vi "MT Generate Bits (Galois, PN Order).vi"(0 "total bits (128)":i32=128, 7 "PN sequence order (9)":i32=9, 9 "seed in (0xD6BF7DF2)":i32=-692093454 format="%.0x", 11 "error in (no error)":errorcluster, 13 "reset? (T)":bool=TRUE) -> (4 "output bit stream":i8[](array[numeric]), 10 "seed out":i32 format="%.0x", 15 "error out":errorcluster)   [LabVIEW 2020, in "niDMT.lvlib"]
doc: "This polymorphic instance generates Galois pseudonoise (PN) bit sequences. The VI repeats the selected pattern until it generates number of total bits that you specify. Use this instance to specify a PN sequence order based on which the VI selects a primitive polynomial that returns an m-sequence."
uses:
  <vilib>/addons/Modulation/niDMT.lvlib
  <vilib>/addons/Modulation/niAMT.lvlib
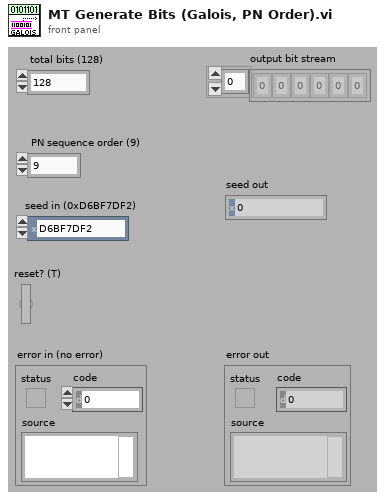
[diagram p1: front panel]
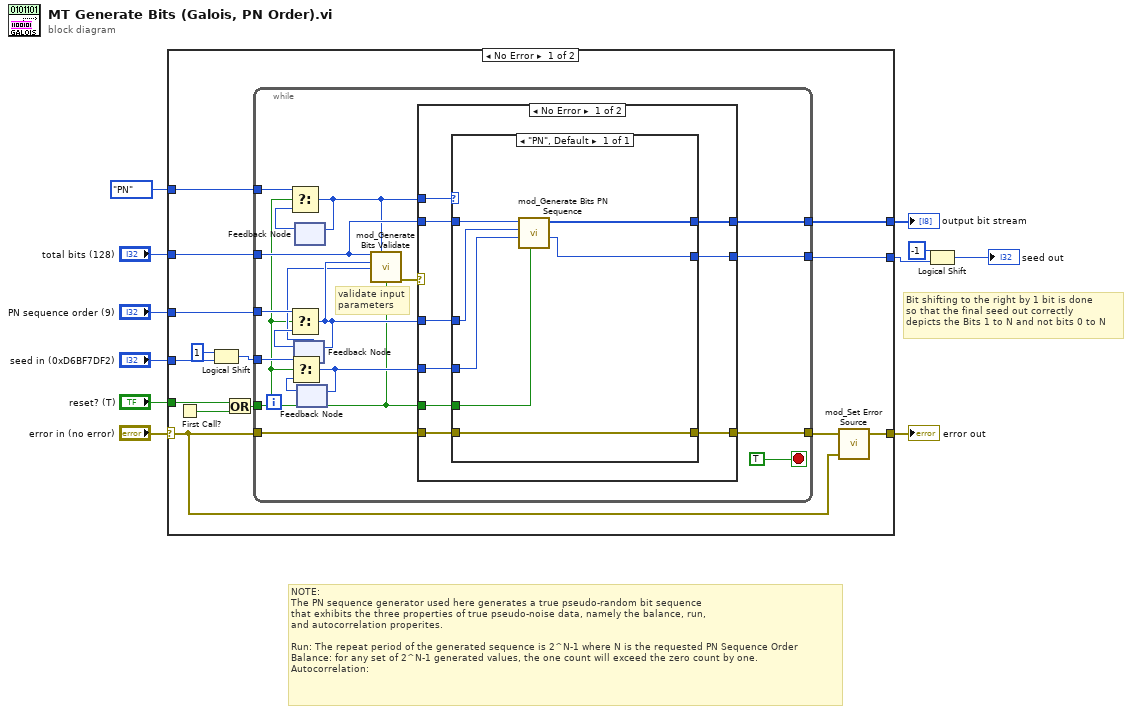
[diagram p0: block diagram]
diagram:
  # "Bit shifting to the right by 1 bit is done \nso that the final seed out correctly \ndepicts the Bits 1 to N and not bits 0 to N"
  # "NOTE:\nThe PN sequence generator used here generates a true pseudo-random bit sequence\nthat exhibits the three properties of true pseudo-noise data, namely the balance, run,\nand autocorrelation properites.\n\nRun: The repeat period of the generated sequence is 2^N-1 where N is the requested PN Sequence Order\nBalance: for any set of 2^N-1 generated values, the one count will exceed the zero count by one.\nAutocorrelation:"
  n1 = case shown="No Error" "error in (no error)" {
    selector: "error in (no error)" -> [w16 w64]
    tunnel: [w21 w64] -> w10
    tunnel: "total bits (128)" -> [w24 _]
    tunnel: enum16{"PN", "pattern", "user"}."PN" ("mode (PN)") -> [w23 _]
    tunnel: "reset? (T)" -> [w18 _]
    tunnel: "seed in (0xD6BF7DF2)" -> [w13 w63]
    tunnel: "PN sequence order (9)" -> [w14 _]
    tunnel: [w25 i8[] []] -> w4
    tunnel: [w20 w63] -> w1
    frame No Error {
      n2 = First Call?() -> (First Call?: T/F=w19:bool)
      n3 = Logical Shift(y=1, x=w13) -> (x << y=w12:i32)
      n4 = Or(x=w18, y=w19) -> (x .or. y?=w17:bool)
      n5 = while {
        tunnel: [w42] -> w25
        tunnel: w24 -> [w33]
        tunnel: w14 -> [w35]
        tunnel: w23 -> [w29]
        tunnel: [w40] -> w22
        tunnel: w16 -> [w39]
        tunnel: [w38] -> w20
        tunnel: w12 -> [w32]
        tunnel: w17 -> [w28]
        stop <- TRUE stop-if-true
        # "validate input parameters"
        n6 = feedback #1() -> (w36:i32)  [unwired: 1 out]
        n7 = Select(t=w35, s=w28, f=w36) -> (s? t:f=w34:i32)
        n8 = feedback-in #1(w34) -> ()
        n9 = feedback #2() -> (w27:enum16{"PN", "pattern", "user"})  [unwired: 1 out]
        n10 = Select(t=w29, s=w28, f=w27) -> (s? t:f=w26:enum16{"PN", "pattern", "user"})
        n11 = feedback-in #2(w26) -> ()
        n12 = feedback #3() -> (w31:i32)  [unwired: 1 out]
        n13 = Select(t=w32, s=w28, f=w31) -> (s? t:f=w30:i32)
        n14 = feedback-in #3(w30) -> ()
        n15 = call <vilib>:"mod_Generate Bits Validate.vi"("Total Bits"=w33, "Mode (PN)"=w26, "PN Sequence Order"=w34, "seed in"=w30, "reset?"=w28) -> ("error out"=w41:errorcluster)  [unwired: 1 in, 9 out]
        n16 = case shown="No Error" w41 {
          selector: w41 -> [_ w61]
          tunnel: w39 -> [w51 _]
          tunnel: [w50 w61] -> w40
          tunnel: w26 -> [w49 _]
          tunnel: [w48 i8[] [] ("Output Data Bit Sequence")] -> w42
          tunnel: w33 -> [w47 _]
          tunnel: w34 -> [w46 _]
          tunnel: w30 -> [w45 w60]
          tunnel: w28 -> [w44 _]
          tunnel: [w43 w60] -> w38
          frame No Error {
            n17 = case shown="\"PN\", Default" w49 {
              tunnel: w51 -> [w55]
              tunnel: [w55] -> w50
              tunnel: [w58] -> w48
              tunnel: w47 -> [w57]
              tunnel: w46 -> [w53]
              tunnel: w45 -> [w52]
              tunnel: w44 -> [w56]
              tunnel: [w54] -> w43
              frame "PN", Default {
                n18 = call <vilib>:"mod_Generate Bits PN Sequence.vi"("Reset? (T)"=w56, "seed in (0xD6BF7DF2)"=w52, "PN Sequence Order (9)"=w53, "Total Bits"=w57) -> ("seed out"=w54:u32, "Output Bit Stream"=w58:i8[])  [unwired: 6 out]
              }
            }
          }
          frame Error {
            # "Invalid inputs - generate error"
          }
        }
      }
      n19 = call <vilib>:"mod_Set Error Source.vi"("initial error in (no error)"=w16, "final error in (no error)"=w22) -> ("error out"=w21:errorcluster)  [unwired: 3 out]
    }
    frame Error {
    }
  }
  "error out" <- w10
  "output bit stream" <- w4
  n20 = Logical Shift(y=-1, x=w1) -> (x << y=→"seed out":u32)
